vi "Thev-Find Fq.vi"(0 "Frequency (Hz)":dbl[](array[numeric]), 5 "Px":cdb[](array[numeric]), 7 "Fmin":dbl=500.0, 9 "Fmax":dbl=10000.0) -> (8 "Fq (Hz)":dbl)   [LabVIEW 2015]
uses:
  <vilib>/Analysis/baseanly.llb/Mean (DBL).vi
  <vilib>/Analysis/NI_AALBase.lvlib
panel:
  out "XY Graph":cluster{"Frequency (Hz)":dbl[], dbl[]}[](graph)
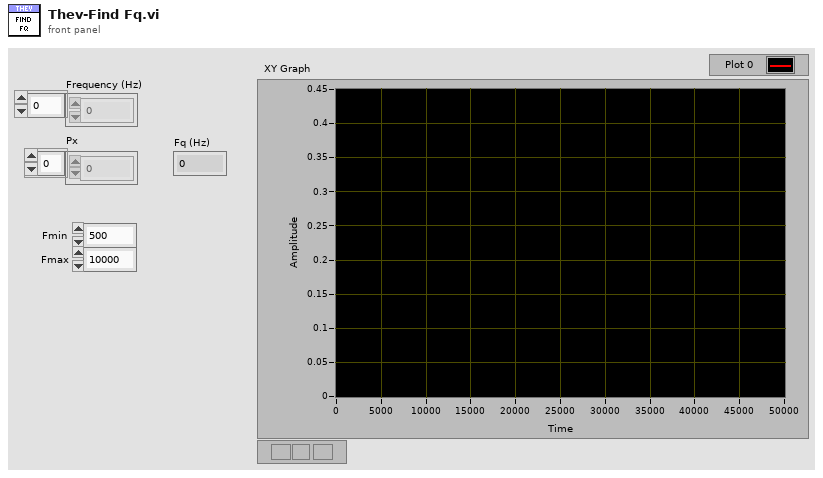
[diagram p1: front panel]
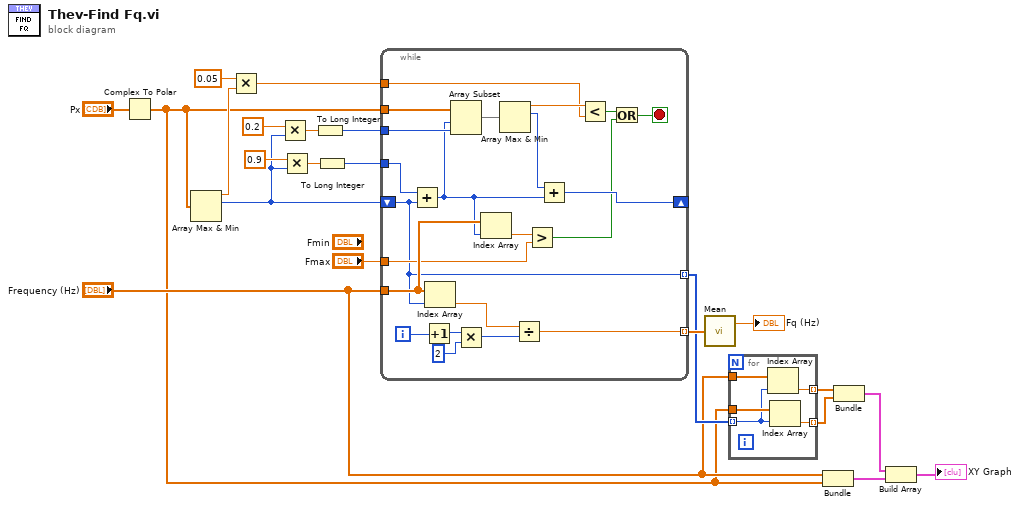
[diagram p0: block diagram]
diagram:
  n1 = Complex To Polar(r * e^(i*theta)="Px") -> (r=w6:dbl[])  [unwired: 1 out]
  n2 = Array Max & Min(array=w6) -> (max value=w22:dbl, max index (indices)=w13:i32)  [unwired: 2 out]
  n3 = Multiply(x=0.05, y=w22) -> (x*y=w14:dbl)
  n4 = Multiply(x=0.2, y=w13) -> (x*y=w19:dbl)
  n5 = Multiply(x=0.9, y=w13) -> (x*y=w17:dbl)
  n6 = To Long Integer(number=w19) -> (32bit integer=w16:i32)
  n7 = To Long Integer(number=w17) -> (32bit integer=w15:i32)
  n8 = while {
    shift-right: [w29] -> _
    shift-left: w13 -> [w23]
    tunnel: w16 -> [w43]
    tunnel: w15 -> [w42]
    tunnel: w6 -> [w44]
    tunnel: w14 -> [w33]
    tunnel: "Frequency (Hz)" -> [w28]
    tunnel: [w39] -> w11 mode=indexing
    tunnel: "Fmax" -> [w25]
    tunnel: [w23] -> w8 mode=indexing
    i -> [w38]
    stop <- w31 stop-if-true
    n9 = Add(x=w42, y=w23) -> (x+y=w27:i32)
    n10 = Increment(x=w38) -> (x+1=w37:i32)
    n11 = Index Array(array=w28, index=w23) -> (element=w30:dbl)
    n12 = Array Subset(array=w44, index=w27, length=w43) -> (w41:dbl[])
    n13 = Multiply(x=w37, y=2) -> (x*y=w35:i32)
    n14 = Index Array(array=w28, index=w27) -> (element=w26:dbl)
    n15 = Array Max & Min(array=w41) -> (max value=w34:dbl, max index (indices)=w40:i32)  [unwired: 2 out]
    n16 = Divide(x=w30, y=w35) -> (x/y=w39:dbl)
    n17 = Greater?(x=w26, y=w25) -> (0:w24:bool)
    n18 = Add(x=w40, y=w27) -> (x+y=w29:i32)
    n19 = Less?(x=w34, y=w33) -> (x < y?=w32:bool)
    n20 = Or(x=w32, y=w24) -> (x .or. y?=w31:bool)
  }
  n21 = call-poly <vilib>:"Mean.vi"("X"=w11) -> ("mean"=→"Fq (Hz)":dbl)  [unwired: 1 out]
  n22 = for {
    tunnel: w8 -> [w47] mode=indexing
    tunnel: "Frequency (Hz)" -> [w49]
    tunnel: w6 -> [w48]
    tunnel: [w46] -> w5 mode=indexing
    tunnel: [w45] -> w4 mode=indexing
    n23 = Index Array(array=w49, index=w47) -> (element=w46:dbl)
    n24 = Index Array(array=w48, index=w47) -> (element=w45:dbl)
  }
  n25 = Bundle("Frequency (Hz)"="Frequency (Hz)", w6) -> (w9:cluster{"Frequency (Hz)":dbl[], dbl[]})  [unwired: 1 in]
  n26 = Bundle(w5, w4) -> (w2:cluster{dbl[], dbl[]})  [unwired: 1 in]
  n27 = Build Array(w2, w9) -> (→"XY Graph":cluster{"Frequency (Hz)":dbl[], dbl[]}[])
